vi "stateMachine.vi"() -> ()   [LabVIEW 2020]
panel:
  out "Temp PV":dbl format="%#.2g"
  out "Waveform Chart":dbl(graph)
  out "x-y":dbl
  out "Power LED":bool
  in  "Play Button":bool
  in  "Temp":dbl
  in  "Time":dbl
  in  "Stop Button":bool
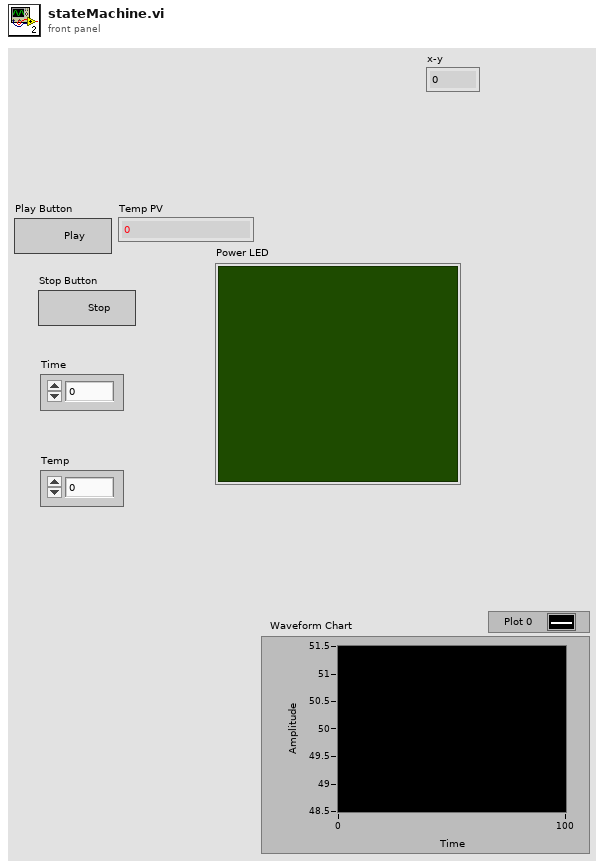
[diagram p1: front panel]
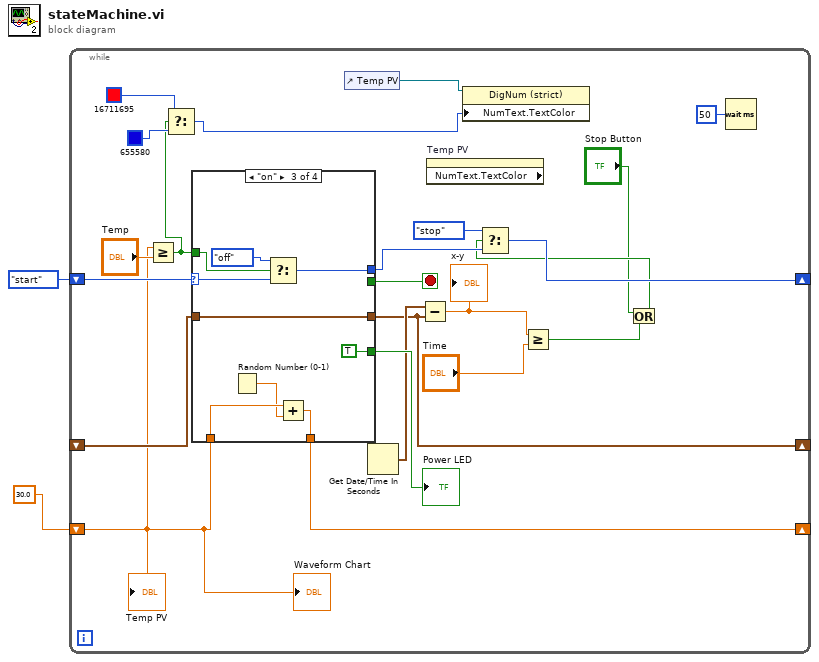
[diagram p0: block diagram]
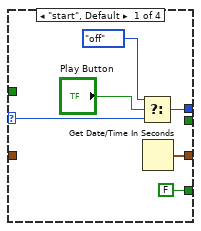
[diagram p2: hidden frame]
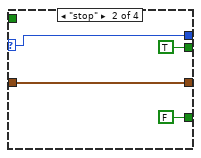
[diagram p3: hidden frame]
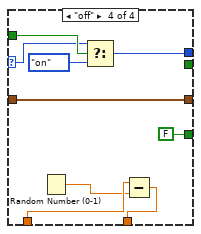
[diagram p4: hidden frame]
diagram:
  n1 = while {
    shift-right: [w13] -> _
    shift-left: enum16{"start", "stop", "on", "off"}."start" -> [w25]
    shift-right: [w19] -> _
    shift-left: _ -> [w21]
    shift-right: [w10] -> _
    shift-left: 30.0 -> [w8]
    stop <- w22 stop-if-true
    n2 = Greater Or Equal?(x=w8, y="Temp") -> (x >= y?=w5:bool)
    n3 = Select(t=u32 16711695 ("Numeric Text.Text Colors:Text Color"), s=w5, f=u32 655580 ("Numeric Text.Text Colors:Text Color")) -> (s? t:f=w3:u32)
    n4 = case shown="\"on\"" w25 {
      selector: w25 -> [w30 w34 w42 w51]
      tunnel: [w29 w34 w40 w49] -> w15
      tunnel: [FALSE FALSE TRUE FALSE] -> w24
      tunnel: w5 -> [_ _ w43 w52]
      tunnel: [_ TRUE _ _] -> w22
      tunnel: [w26 w32 w39 w48] -> w19
      tunnel: w21 -> [_ w32 w39 w48]
      tunnel: w8 -> [_ _ w38 w47]
      tunnel: [_ _ w36 w45] -> w10
      frame "start", Default {
        n5 = Select(t=enum16{"start", "stop", "on", "off"}."off", s="Play Button", f=w30) -> (s? t:f=w29:enum16{"start", "stop", "on", "off"})
        n6 = Get Date/Time In Seconds() -> (seconds since 1Jan1904=w26:timestamp)
      }
      frame "stop" {
      }
      frame "on" {
        n7 = Random Number (0-1)() -> (number: 0 to 1=w37:dbl)
        n8 = Select(t=enum16{"start", "stop", "on", "off"}."off", s=w43, f=w42) -> (s? t:f=w40:enum16{"start", "stop", "on", "off"})
        n9 = Add(x=w38, y=w37) -> (x+y=w36:dbl)
      }
      frame "off" {
        n10 = Random Number (0-1)() -> (number: 0 to 1=w46:dbl)
        n11 = Select(t=w51, s=w52, f=enum16{"start", "stop", "on", "off"}."on") -> (s? t:f=w49:enum16{"start", "stop", "on", "off"})
        n12 = Subtract(x=w47, y=w46) -> (x-y=w45:dbl)
      }
    }
    "Power LED" <- w24
    n13 = control-ref of="Temp PV"() -> (w4:refnum<vi>)
    n14 = Get Date/Time In Seconds() -> (seconds since 1Jan1904=w20:timestamp)
    n15 = Subtract(x=w20, y=w19) -> (x-y=w18:dbl)
    "x-y" <- w18
    n16 = property on="Temp PV" class="DigNum (strict)" props=["NumText", "TextColor"]() -> ()  [unwired: 2 in, 3 out]
    n17 = property class="DigNum (strict)"(reference=w4, "NumText.TextColor"=w3) -> ()  [unwired: 1 in, 2 out]
    n18 = Greater Or Equal?(x=w18, y="Time") -> (x >= y?=w16:bool)
    n19 = Or(x="Stop Button", y=w16) -> (x .or. y?=w12:bool)
    n20 = Select(t=enum16{"start", "stop", "on", "off"}."stop", s=w12, f=w15) -> (s? t:f=w13:enum16{"start", "stop", "on", "off"})
    n21 = Wait (ms)(milliseconds to wait=u32 50) -> ()  [unwired: 1 out]
    "Waveform Chart" <- w8
    "Temp PV" <- w8
  }
